vi "Clear Follow Record.vi"(9 "Current Choice Index":i32, 11 "Selected Choices":T1[](array[typedef])) -> (3 "Selected Choices Out":T1[](array[typedef]))   [LabVIEW 2021]
uses:
  Control/Answers.ctl
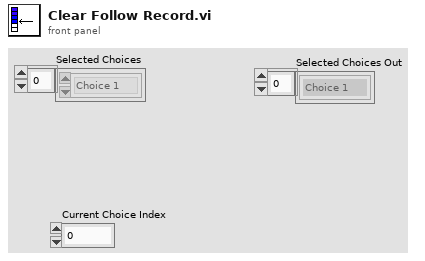
[diagram p1: front panel]
types:
  T1 = typedef "Answers.ctl" = enum16{"Choice 1", "Choice 2"}
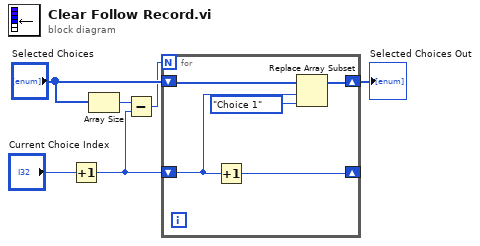
[diagram p0: block diagram]
diagram:
  n1 = Increment(x="Current Choice Index") -> (x+1=w2:i32)
  n2 = Array Size(array="Selected Choices") -> (size(s)=w3:i32)
  n3 = Subtract(x=w3, y=w2) -> (x-y=w1:i32)
  n4 = for {
    N: w1 -> [_]
    shift-right: [w9] -> w4
    shift-left: "Selected Choices" -> [w11]
    shift-right: [w7] -> _
    shift-left: w2 -> [w8]
    n5 = Increment(x=w8) -> (x+1=w7:i32)
    n6 = Replace Array Subset(array=w11, new element=Answers."Choice 1" ("new element/subarray"), index=w8) -> (w9:T1[])
  }
  "Selected Choices Out" <- w4
